vi "Try posix-rename.vi"(6 "Deadline in":T1, 8 "error in (no error)":errorcluster, 9 "to":string, 10 "from":string, 11 "session in":refnum<class "Session.lvclass">) -> (0 "error out":errorcluster, 3 "session out":refnum<class "Session.lvclass">)   [LabVIEW 2020, in "NI_SFTP.lvlib"]
uses:
  <vilib>/net/SFTP/NI_SFTP.lvlib
  <vilib>/Utility/Deadline/Deadline.ctl
  <vilib>/Utility/Deadline/Mode.ctl
  <vilib>/net/SFTP/Session/Session.lvclass
  <vilib>/net/SFTP/API/Support/Command/posix-rename_openssh.com/Input.ctl
  <vilib>/net/SFTP/API/Support/Command/posix-rename_openssh.com/posix-rename_openssh.com.lvclass
  <vilib>/Utility/Deadline/NI_Deadline.lvlib
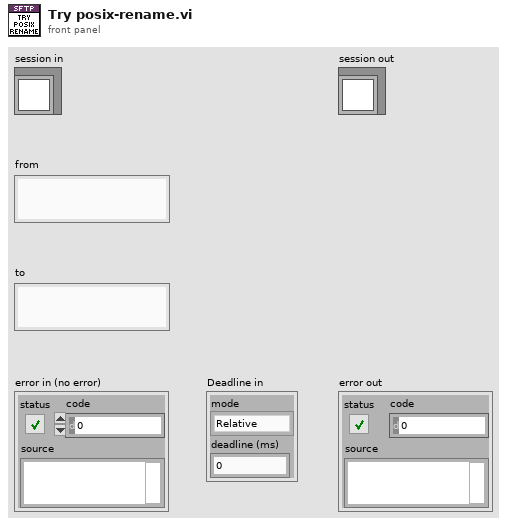
[diagram p1: front panel]
types:
  T1 = typedef "NI_Deadline.lvlib/Deadline.ctl" = cluster{"mode":T2, "deadline (ms)":u32}
  T2 = typedef "NI_Deadline.lvlib/Mode.ctl" = enum16{"Relative", "Use deadline", "Wait forever", "Nonblocking", "N/A"}
  T3 = typedef "NI_SFTP.lvlib/posix-rename_openssh.com.lvclass/Input.ctl" = cluster{"from":string, "to":string}
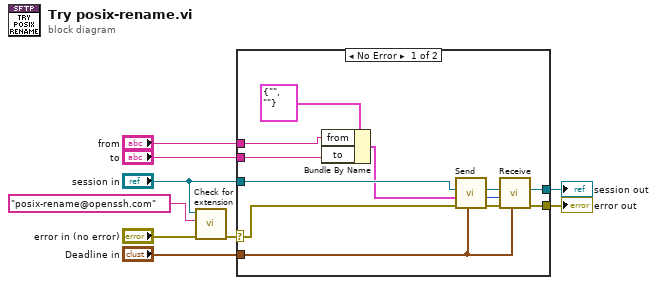
[diagram p0: block diagram]
diagram:
  n1 = call <vilib>:"Check for extension.vi"("error in (no error)"="error in (no error)", "extension name"="posix-rename@openssh.com" ("name"), "session in"="session in") -> ("error out"=w1:errorcluster)  [unwired: 8 in]
  n2 = case shown="No Error" w1 {
    selector: w1 -> [w19 w22]
    tunnel: "Deadline in" -> [w21 _]
    tunnel: [w20 w22] -> w8
    tunnel: [w11 w23] -> w7
    tunnel: "session in" -> [w15 w23]
    tunnel: "from" -> [w14 _]
    tunnel: "to" -> [w13 _]
    frame No Error {
      n3 = Bundle By Name(cluster=T3 {"from"="", "to"=""} ("input"), "from"=w14, "to"=w13) -> (w12:T3)
      n4 = call <vilib>:"Send.vi"("Timeout"=w21, "error in (no error)"=w19, "input"=w12, "session in"=w15) -> ("error out"=w18:errorcluster, "request id"=w10:u32, "session out"=w17:refnum<class "Session.lvclass">)  [unwired: 4 in, 1 out]
      n5 = call <vilib>:"Receive.vi"("Timeout"=w21, "error in (no error)"=w18, "request id"=w10, "session in"=w17) -> ("error out"=w20:errorcluster, "session out"=w11:refnum<class "Session.lvclass">)  [unwired: 4 in, 2 out]
    }
    frame Error {
    }
  }
  "error out" <- w8
  "session out" <- w7
